vi "NI VeriStand - Set Multiple Dependent Node Refs.vi"(8 "error in (no error)":errorcluster, 9 "Dependent Node Refs":T1[](array[typedef]) format="%.0x", 10 "Base Property Name":string, 11 "Item Ref in":T1 format="%.0x") -> (0 "error out":errorcluster, 3 "Item Ref out":T1=18446744073709551615 format="%.0x")   [LabVIEW 2020, in "Custom Device Utility Library.lvlib"]
doc: "Sets multiple properties, with dependent node references as values, on a custom device item. Dependent node references map to other nodes in the custom device, such as channels from which properties get their values."
uses:
  <vilib>/NI VeriStand/Custom Device Tools/Custom Device Utility Library/Custom Device Utility Library.lvlib
  <vilib>/NI VeriStand/Custom Device API/Custom Device Item Ref.ctl
  <vilib>/NI VeriStand/Custom Device API/Set Item Property (Dependent Node Pointer).vi
  <vilib>/NI VeriStand/Custom Device API/Custom Device API.lvlib
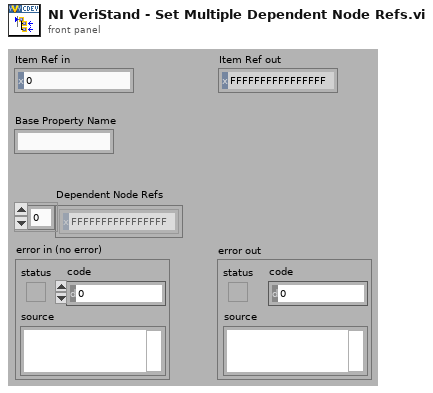
[diagram p1: front panel]
types:
  T1 = typedef "Custom Device API.lvlib/Custom Device Item Ref.ctl" = u64
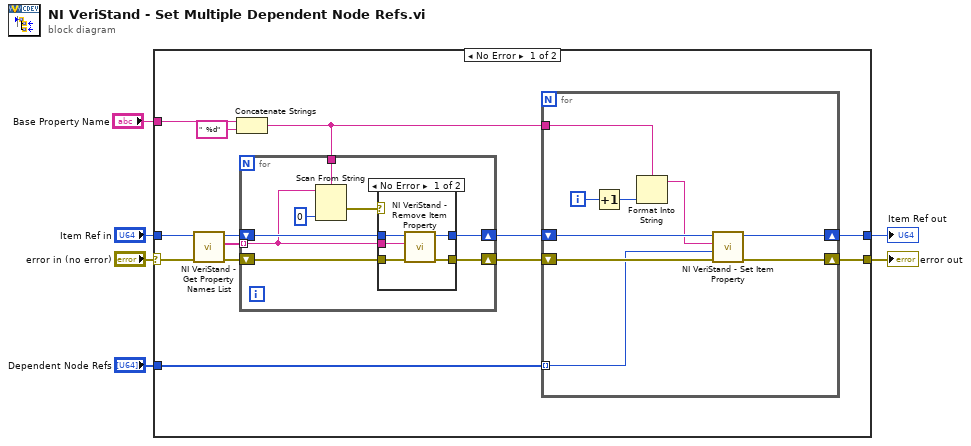
[diagram p0: block diagram]
diagram:
  n1 = case shown="No Error" "error in (no error)" {
    selector: "error in (no error)" -> [w7 w44]
    tunnel: "Item Ref in" -> [w19 w45]
    tunnel: "Dependent Node Refs" -> [w13 _]
    tunnel: [w12 w45] -> w4
    tunnel: [w11 w44] -> w3
    tunnel: "Base Property Name" -> [w10 _]
    frame No Error {
      n2 = call <vilib>:"NI VeriStand - Get Property Names List.vi"("error in (no error)"=w7, "Item Ref in"=w19) -> ("error out"=w17:errorcluster, "Property Names"=w16:string[], "Item Ref out"=w18:T1)  [unwired: 7 in]
      n3 = Concatenate Strings(w10, "  %d" ("string")) -> (w8:string)
      n4 = for {
        shift-right: [w32] -> w15
        shift-left: w17 -> [w34]
        tunnel: w16 -> [w33] mode=indexing
        shift-right: [w31] -> w14
        shift-left: w18 -> [w36]
        tunnel: w8 -> [w30]
        n5 = Scan From String(format string=w30, input string=w33, default 1=0 ("default value 1")) -> (error out=w35:errorcluster)  [unwired: 3 in, 2 out]
        n6 = case shown="No Error" w35 {
          tunnel: w36 -> [w41 w42]
          tunnel: w34 -> [w40 w43]
          tunnel: w33 -> [w39 _]
          tunnel: [w38 w43] -> w32
          tunnel: [w37 w42] -> w31
          frame No Error {
            n7 = call <vilib>:"NI VeriStand - Remove Item Property.vi"("error in (no error)"=w40, "Property Name"=w39, "Item Ref in"=w41) -> ("error out"=w38:errorcluster, "Item Ref out"=w37:T1)  [unwired: 6 in, 1 out]
          }
          frame Error {
          }
        }
      }
      n8 = for {
        shift-right: [w27] -> w11
        shift-left: w15 -> [w28]
        tunnel: w8 -> [w25]
        shift-right: [w23] -> w12
        shift-left: w14 -> [w24]
        tunnel: w13 -> [w21] mode=indexing
        i -> [w26]
        n9 = Increment(x=w26) -> (x+1=w20:i32)
        n10 = Format Into String(format string=w25, w20) -> (resulting string=w22:string)  [unwired: 2 in, 1 out]
        n11 = call-poly <vilib>:"NI VeriStand - Set Item Property.vi"("error in (no error)"=w28, "Dependent Node Ref"=w21, "Property Name"=w22, "Item Ref in"=w24) -> ("error out"=w27:errorcluster, "Item Ref out"=w23:T1)  [unwired: 6 out]
      }
    }
    frame Error {
    }
  }
  "Item Ref out" <- w4
  "error out" <- w3
